vi "Current Write.vi"   [LabVIEW 2023, in "Device.lvclass"]
uses:
  Device.lvclass
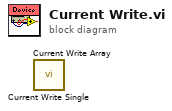
[diagram p0: block diagram]
diagram:
  n1 = call "Current Write Single.vi"() -> ()  [unwired: 11 in, 1 out]
  n2 = call "Current Write Array.vi"() -> ()  [unwired: 11 in, 1 out]
